vi "MotionTest.vi"() -> ()   [LabVIEW 2013]
panel:
  in  "BraggArray":dbl[](array[numeric])
  out "XY Graph":cluster{"X":dbl, "Y":dbl}[](graph)
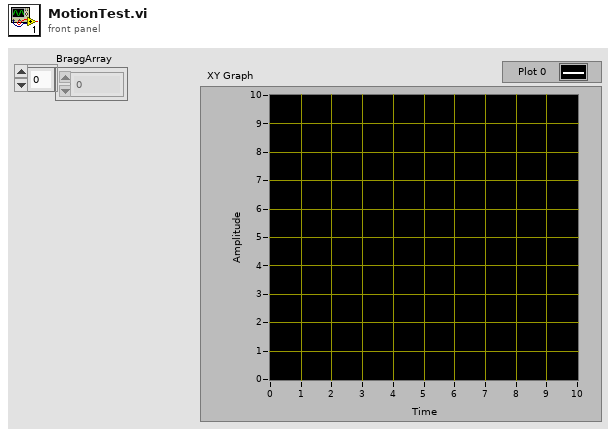
[diagram p1: front panel]
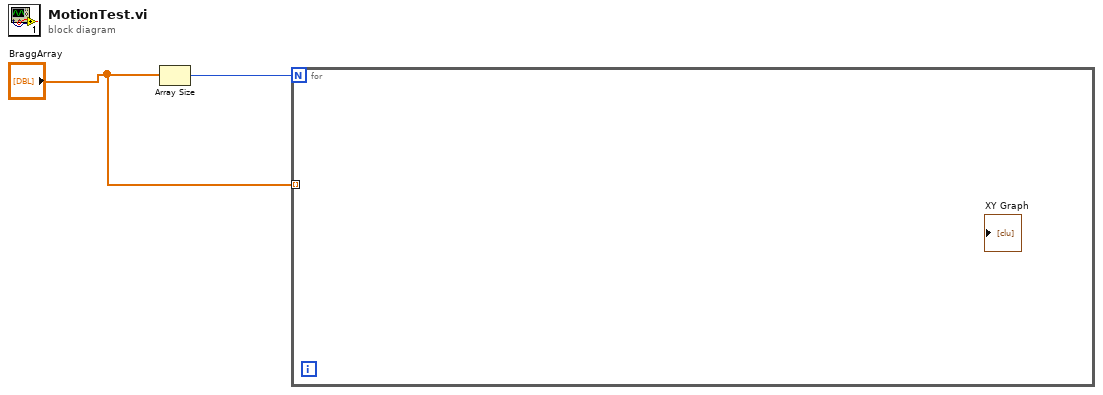
[diagram p0: block diagram]
diagram:
  n1 = Array Size(array="BraggArray") -> (size(s)=w2:i32)
  n2 = for {
    N: w2 -> [_]
    tunnel: "BraggArray" -> [_] mode=indexing
  }
